vi "IO_18v7 Control Algorithm.vi"(6 "error in (no error)":errorcluster, 7 "VISA Refnum in":refnum<visa-resource-name>, 8 "Pump Params":T2 {"RNG_STOP" format="%#_13g"; "RNG_CREEP" format="%#_13g"; "RNG_SLOW" format="%#_13g"}, 9 "Pump Manual Controls":T3, 10 "State Ref":refnum<vi>, 11 "Level SP":dbl(slide)=7.199999999999999 scale=0.0..10.0) -> (1 "Pump Speed Out":T1, 2 "Laser Raw":dbl, 3 "Sim Level":bool, 4 "error out":errorcluster, 5 "VISA Refnum out":refnum<visa-resource-name>)   [LabVIEW 2024]
uses:
  PWC-OLS2/PWC-OLS/PWC-OLS/Control Definitions/Def_PumpSpeed.ctl
  PWC-OLS2/PWC-OLS/PWC-OLS/Control Definitions/DEF_PumpManCtl.ctl
  PWC-OLS2/PWC-OLS/PWC-OLS/Control Definitions/DEF_PumpParams.ctl
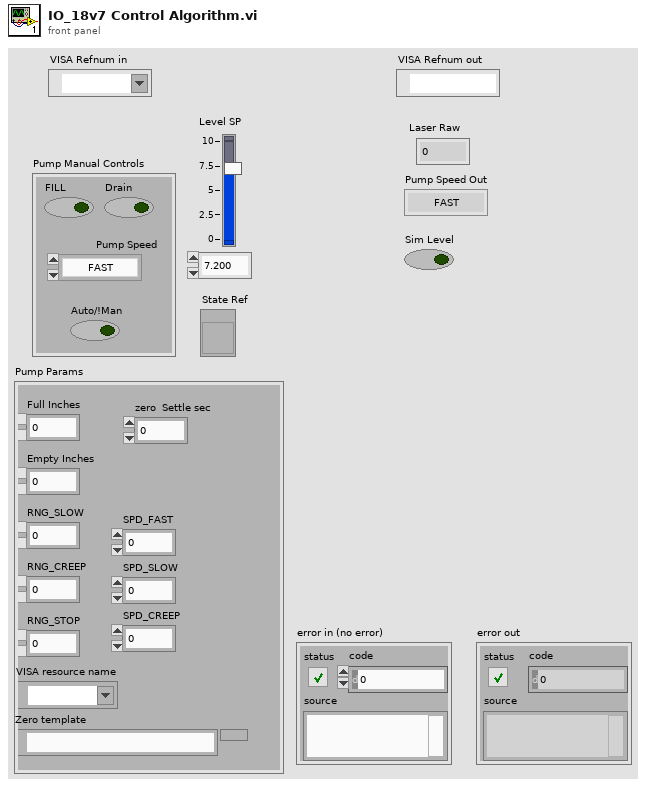
[diagram p1: front panel]
types:
  T1 = typedef "Def_PumpSpeed.ctl" = enum16{"FAST", "SLOW", "CREEP", "STOP"}
  T2 = typedef "DEF_PumpParams.ctl" = cluster{"Empty Inches":dbl, "Full Inches":dbl, "RNG_SLOW":dbl, "RNG_CREEP":dbl, "RNG_STOP ":dbl, "VISA resource name":refnum<visa-resource-name>, "SPD_SLOW":i32, "SPD_CREEP":i32, "SPD_FAST":i32, "Zero template":path, "zero  Settle sec":dbl}
  T3 = typedef "DEF_PumpManCtl.ctl" = cluster{"Pump Speed":T1, "FILL":bool, "Drain":bool, "Auto/!Man":bool}
  T4 = typedef "Def_CalState_Enum.ctl" = enum16{"Start", "Get Info", "Get SP", "Going to SP", "Wait Settle", "Get Measure", "Save Measure", "Done", "Manual"}
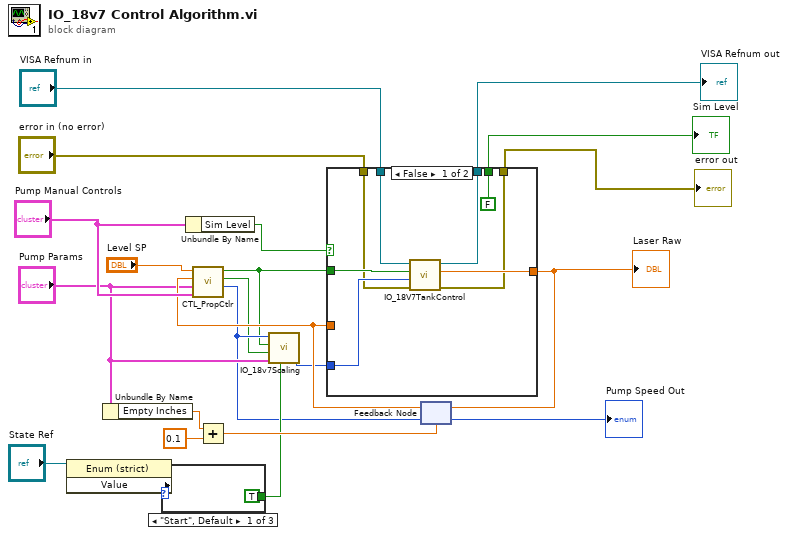
[diagram p0: block diagram]
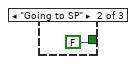
[diagram p2: hidden frame]
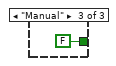
[diagram p3: hidden frame]
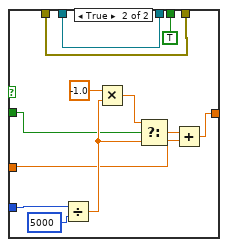
[diagram p4: hidden frame]
diagram:
  n1 = property class="Enum (strict)"(reference="State Ref") -> ("Value"=w11:T4)  [unwired: 1 in, 2 out]
  n2 = Unbundle By Name("Pump Params") -> ("Empty Inches"=w16:dbl)
  n3 = case shown="\"Start\", Default" w11 {
    tunnel: [TRUE FALSE FALSE] -> w12
    frame "Start", Default {
    }
    frame "Going to SP" {
    }
    frame "Manual" {
    }
  }
  n4 = Unbundle By Name("Pump Manual Controls") -> ("Sim Level"=w21:bool)
  n5 = Add(x=w16, y=0.1) -> (x+y=w19:dbl)
  n6 = feedback #1(w19) -> (w18:dbl)
  n7 = call "CTL_PropCtlr.vi"("Pump Manual Controls"="Pump Manual Controls", "Pump Params"="Pump Params", "Level PV"=w18, "Level SP"="Level SP") -> ("Pump Speed Out"=w8:T1, "X< Neg"=w6:bool, "X>Pos"=w7:bool)  [unwired: 4 in, 1 out]
  "Pump Speed Out" <- w8
  n8 = call "IO_18v7Scaling.vi"("!Enabled"=w12, "Pump Params"="Pump Params", "Drain"=w6, "Fill"=w7, "Pump Speed"=w8) -> ("Speed Out"=w9:i32)  [unwired: 5 in, 1 out]
  n9 = case shown="False" w21 {
    tunnel: w18 -> [_ w33]
    tunnel: [w32 w34] -> w17
    tunnel: w7 -> [w31 w35]
    tunnel: w9 -> [w30 w38]
    tunnel: [w29 w40] -> w3
    tunnel: [w28 w39] -> w10
    tunnel: "VISA Refnum in" -> [w27 w40]
    tunnel: "error in (no error)" -> [w26 w39]
    tunnel: [FALSE TRUE] -> w13
    frame False {
      n10 = call "IO_18V7TankControl.vi"("error in"=w26, "Speed"=w30, "Fill!Drain"=w31, "VISA Refnum in"=w27) -> ("error out"=w28:errorcluster, "Laser Raw"=w32:sgl, "VISA Refnum out"=w29:refnum<visa-resource-name>)  [unwired: 4 in, 1 out]
    }
    frame True {
      n11 = Divide(x=w38, y=5000) -> (x/y=w42:dbl)
      n12 = Multiply(x=-1.0 ("y"), y=w42) -> (x*y=w43:dbl)
      n13 = Select(t=w43, s=w35, f=w42) -> (s? t:f=w37:dbl)
      n14 = Add(x=w37, y=w33) -> (x+y=w34:dbl)
    }
  }
  "Laser Raw" <- w17
  "Sim Level" <- w13
  "error out" <- w10
  "VISA Refnum out" <- w3
  n15 = feedback-in #1(w17) -> ()
